vi "SensorsToDash.vi"(0 "Gyro1":dbl, 1 "Name(Sensors)":string="Sensors", 5 "Gyro1Raw":dbl, 7 "Pot1":dbl, 9 "Pot1Raw":dbl, 11 "error in (no error)":errorcluster) -> (15 "error out":errorcluster)   [LabVIEW 2012]
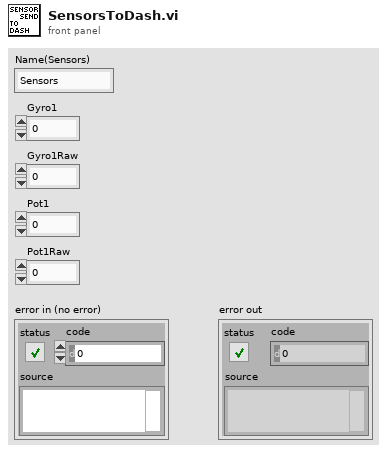
[diagram p1: front panel]
types:
  T1 = cluster{"Gyro1":dbl, "Gyro1Raw":dbl, "Pot1":dbl, "Pot1Raw":dbl}
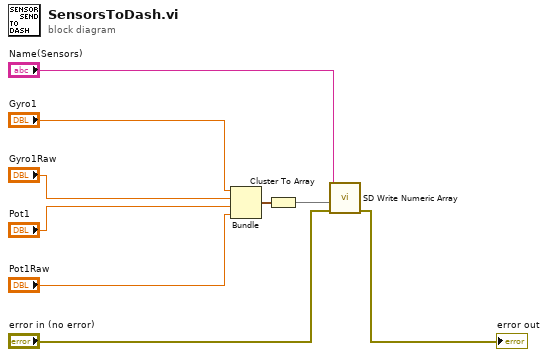
[diagram p0: block diagram]
diagram:
  n1 = Bundle("Gyro1"="Gyro1", "Gyro1Raw"="Gyro1Raw", "Pot1"="Pot1", "Pot1Raw"="Pot1Raw") -> (w5:T1)  [unwired: 1 in]
  n2 = Cluster To Array(cluster=w5) -> (array=w4:dbl[])
  n3 = call <vilib>:"SD Write Numeric Array.vi"("error in"="error in (no error)", "Numeric Array"=w4, "Name"="Name(Sensors)") -> ("error out"=→"error out":errorcluster)  [unwired: 7 in, 1 out]
